vi "publish -- get -- 7.vi"(8 "request event":refnum<user-event>, 9 "response ref":refnum<vi>) -> (2 "nnumber":dbl=1000.0 format="%#_10f")   [LabVIEW 2018]
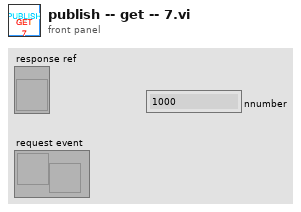
[diagram p1: front panel]
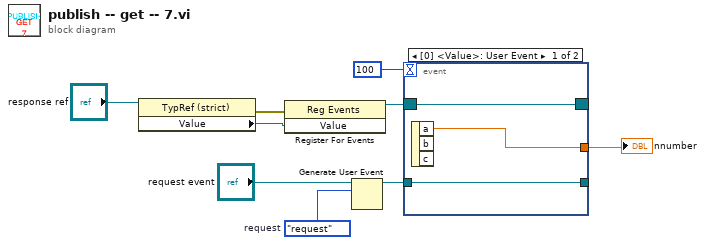
[diagram p0: block diagram]
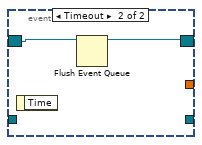
[diagram p2: hidden frame]
diagram:
  w9 = enum16{"request"}."request"  # request
  n1 = property class="TypRef (strict)"(reference="response ref") -> (error out=w3:errorcluster, "Value"=w1:refnum<user-event>)  [unwired: 1 in, 1 out]
  n2 = register-events(error in=w3, w1) -> (reference out=w5:refnum<event-registration>)  [unwired: 1 in, 1 out]
  n3 = Generate User Event(user event="request event", event data cluster=w9) -> (user event out=w6:refnum<user-event>)  [unwired: 2 in, 1 out]
  n4 = event shown="[0] <Value>: User Event" {
    selector: w5 -> [w10 w14]
    dyn-events: [w10 w13] -> _
    timeout: 100 -> [_ _]
    tunnel: [w12 _] -> w8
    tunnel: [w11 _] -> _
    tunnel: w6 -> [w11 _]
    event User Event {
      n5 = event-data() -> ("a"=w12:dbl)  [unwired: 1 in, 2 out]
    }
    event Timeout {
      n6 = event-data() -> ()  [unwired: 1 in, 1 out]
      n7 = Flush Event Queue(0:w14) -> (8:w13:refnum<event-registration>)  [unwired: 5 in, 2 out]
    }
  }
  "nnumber" <- w8
